vi "Get Type.vi"(8 "error in (no error)":errorcluster, 11 "DBL Connection in":refnum<class "DBL Connection.lvclass">) -> (0 "error out":errorcluster, 2 "Type":T1, 3 "DBL Connection out":refnum<class "DBL Connection.lvclass">)   [LabVIEW 2020, in "Parallel Block.lvlib" / "DBL Connection.lvclass"]
uses:
  DBL Connection.lvclass
  Value Type.ctl
  DBL Connection.lvclass/DBL Connection.ctl
  Parallel Block.lvlib
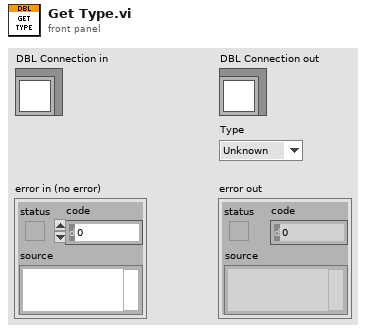
[diagram p1: front panel]
types:
  T1 = typedef "Parallel Block.lvlib/Value Type.ctl" = enum16{"Unknown", "Bool", "U8", "U16", "U32", "U64", "I8", "I16", "I32", "I64", "SGL", "DBL", "CSG", "CDB", "CDBWfm", "String", "DBLWfm"}
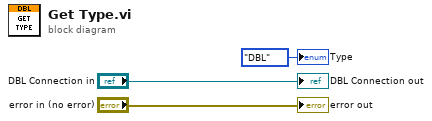
[diagram p0: block diagram]
diagram:
  "error out" <- "error in (no error)"
  "DBL Connection out" <- "DBL Connection in"
  "Type" <- Value_Type."DBL" ("Type")
